vi "logForceActuatorSafetyCheck.vi"(8 "error in (no error)":errorcluster, 10 "EventForceActuatorSafetyChecks":T1, 11 "M1M3SAL in":refnum<class "M1M3SAL.lvclass">) -> (0 "error out":errorcluster, 3 "M1M3SAL out":refnum<class "M1M3SAL.lvclass">)   [LabVIEW 2016, in "M1M3SupportCommunicator.lvlib" / "M1M3SAL.lvclass"]
uses:
  M1M3SAL.lvclass
  DataTypes/Topics/EventForceActuatorSafetyChecks.ctl
  DataTypes/Topics/Parts/Timestamp.ctl
  DataTypes/MessageHeader.ctl
  DataTypes/MessageTypes.ctl
  DataTypes/MessageTopics.ctl
  Common_RT_Utilities/U8ArrayBuilderAutoIndexing/U8ArrayBuilderAutoIndexing.lvclass
  M1M3SupportCommunicator.lvlib
  DataTypes/Topics/M1M3SupportTopics.lvlib
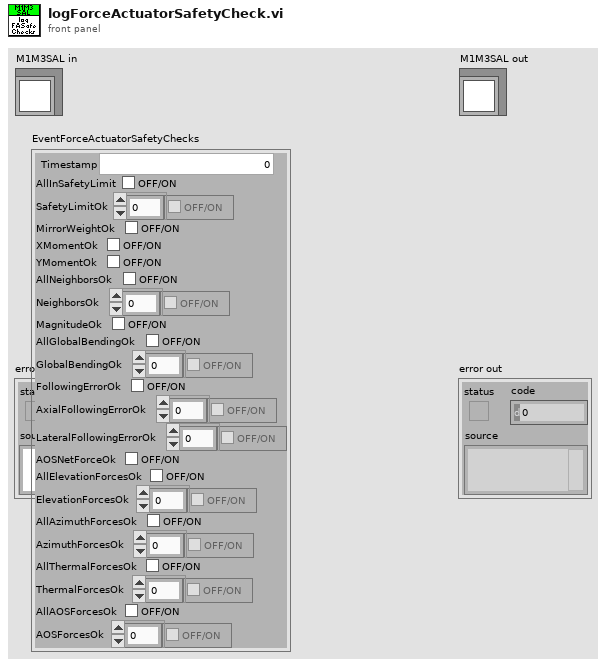
[diagram p1: front panel]
types:
  T1 = typedef "M1M3SupportTopics.lvlib/EventForceActuatorSafetyChecks.ctl" = cluster{"Timestamp":T2, "AllInSafetyLimit":bool, "SafetyLimitOk":bool[], "MirrorWeightOk":bool, "XMomentOk":bool, "YMomentOk":bool, "AllNeighborsOk":bool, "NeighborsOk":bool[], "MagnitudeOk":bool, "AllGlobalBendingOk":bool, "GlobalBendingOk":bool[], "FollowingErrorOk":bool, "AxialFollowingErrorOk":bool[], "LateralFollowingErrorOk":bool[], "AOSNetForceOk":bool, "AllElevationForcesOk":bool, "ElevationForcesOk":bool[], "AllAzimuthForcesOk":bool, "AzimuthForcesOk":bool[], "AllThermalForcesOk":bool, "ThermalForcesOk":bool[], "AllAOSForcesOk":bool, "AOSForcesOk":bool[]}
  T2 = typedef "M1M3SupportTopics.lvlib/Timestamp.ctl" = dbl
  T3 = typedef "M1M3SupportCommunicator.lvlib/MessageHeader.ctl" = cluster{"Type":T4, "Topic":T5, "Size":i32}
  T4 = typedef "M1M3SupportCommunicator.lvlib/MessageTypes.ctl" = enum8{"None", "PutSample", "GetNextSample", "LogEvent", "GetEvent", "IssueCommand", "CommandId", "WaitForCompletion", "AcceptCommand", "AckCommand"}
  T5 = typedef "M1M3SupportCommunicator.lvlib/MessageTopics.ctl" = enum8{"None", "ForceActuatorData", "MirrorForceData", "HardpointData", "AirData", "DynamicData", "FPGAData", "IMSData", "ForceActuatorStatus", "ElevationData", "HardpointStatus", "HardpointActuatorChase", "AirStatus", "ForceActuatorSafetyChecks", "ForceActuatorTest", "ActuatorBroadcastCounter", "StatusChecks", "CellChecks", "HardpointActuatorBreakaway", "RaiseMirrorComplete", "ILCCommunication", "ElevationAngleChecks", "DetailedState", "ServoLoops", "ForceActuatorInfo", "LowerMirrorComplete", "HardpointActuatorInfo", "SettingsApplied", "ErrorCode", "StartupChecks", "SummaryState", "SettingVersions", "ActuatorTestStatus", "AppliedSettingsMatchStart", "Enable", "EnterMaintenance", "Standby", "AbortLowerM1M3", "ApplyAberrationByForces", "ApplyAOSCorrectionByBendingModes", "ClearAOSCorrection", "Start", "RaiseM1M3", "TestForceActuator", "LowerM1M3", "ApplyAOSCorrectionByForces", "Disable", "ApplyAberationByBendingMode", "TestHardpoint", "ManipulateM1M3", "ClearAberration", "Exit", "TestAir", "AbortRaiseM1M3", "MoveHardpointActuators", "ExitMaintenance", "Shutdown"}
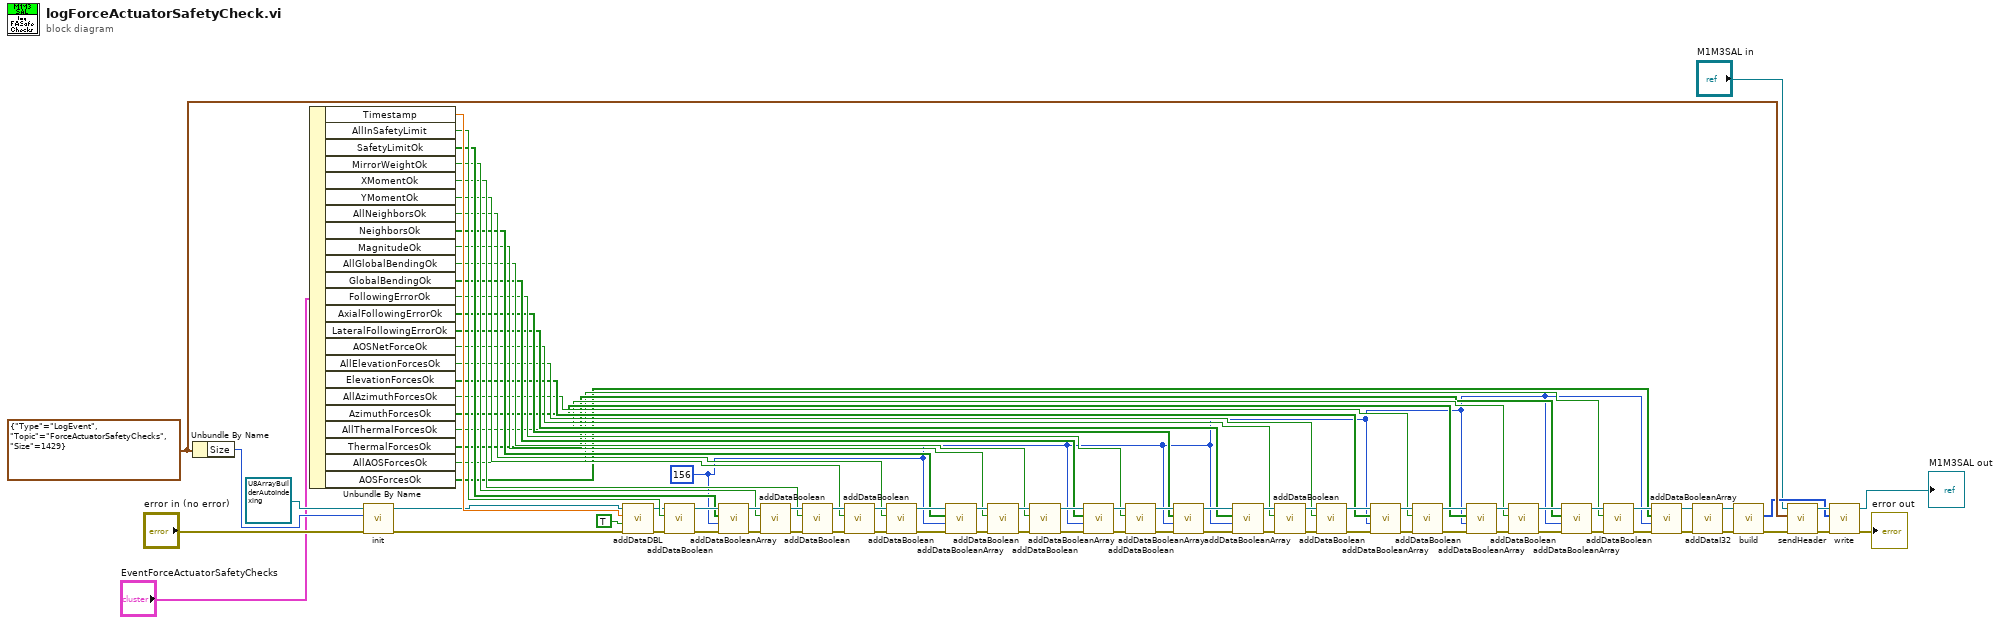
[diagram p0: block diagram]
diagram:
  w1 = 156 ("Length")
  w86 = T3 {"Type"=enum."LogEvent", "Topic"=enum."ForceActuatorSafetyChecks", "Size"=1429} ("MessageHeader")
  n1 = Unbundle By Name(w86) -> ("Size"=w85:i32)
  n2 = Unbundle By Name("EventForceActuatorSafetyChecks") -> ("Timestamp"=w76:T2, "AllInSafetyLimit"=w29:bool, "SafetyLimitOk"=w28:bool[], "MirrorWeightOk"=w27:bool, "XMomentOk"=w26:bool, "YMomentOk"=w25:bool, "AllNeighborsOk"=w24:bool, "NeighborsOk"=w23:bool[], "MagnitudeOk"=w22:bool, "AllGlobalBendingOk"=w21:bool, "GlobalBendingOk"=w20:bool[], "FollowingErrorOk"=w19:bool, "AxialFollowingErrorOk"=w18:bool[], "LateralFollowingErrorOk"=w17:bool[], "AOSNetForceOk"=w16:bool, "AllElevationForcesOk"=w15:bool, "ElevationForcesOk"=w14:bool[], "AllAzimuthForcesOk"=w13:bool, "AzimuthForcesOk"=w12:bool[], "AllThermalForcesOk"=w11:bool, "ThermalForcesOk"=w10:bool[], "AllAOSForcesOk"=w9:bool, "AOSForcesOk"=w8:bool[])
  n3 = call "init.vi"("error in (no error)"="error in (no error)", "Size"=w85, "U8ArrayBuilderAutoIndexing in"=refnum<class "U8ArrayBuilderAutoIndexing.lvclass"> refnum ("RTUtilities.lvlib:U8ArrayBuilderAutoIndexing.lvclass")) -> ("error out"=w73:errorcluster, "U8ArrayBuilderAutoIndexing out"=w75:refnum<class "U8ArrayBuilderAutoIndexing.lvclass">)  [unwired: 7 in]
  n4 = call "addDataDBL.vi"("error in (no error)"=w73, "OverrideSwapBytes"=TRUE, "Data"=w76, "U8ArrayBuilderAutoIndexing in"=w75) -> ("error out"=w6:errorcluster, "U8ArrayBuilderAutoIndexing out"=w7:refnum<class "U8ArrayBuilderAutoIndexing.lvclass">)  [unwired: 6 in]
  n5 = call "addDataBoolean.vi"("error in (no error)"=w6, "Data"=w29, "U8ArrayBuilderAutoIndexing in"=w7) -> ("error out"=w34:errorcluster, "U8ArrayBuilderAutoIndexing out"=w35:refnum<class "U8ArrayBuilderAutoIndexing.lvclass">)  [unwired: 7 in]
  n6 = call "addDataBooleanArray.vi"("error in (no error)"=w34, "Length"=w1, "Data"=w28, "U8ArrayBuilderAutoIndexing in"=w35) -> ("error out"=w71:errorcluster, "U8ArrayBuilderAutoIndexing out"=w70:refnum<class "U8ArrayBuilderAutoIndexing.lvclass">)  [unwired: 6 in]
  n7 = call "addDataBoolean.vi"("error in (no error)"=w71, "Data"=w27, "U8ArrayBuilderAutoIndexing in"=w70) -> ("error out"=w69:errorcluster, "U8ArrayBuilderAutoIndexing out"=w68:refnum<class "U8ArrayBuilderAutoIndexing.lvclass">)  [unwired: 7 in]
  n8 = call "addDataBoolean.vi"("error in (no error)"=w69, "Data"=w26, "U8ArrayBuilderAutoIndexing in"=w68) -> ("error out"=w67:errorcluster, "U8ArrayBuilderAutoIndexing out"=w66:refnum<class "U8ArrayBuilderAutoIndexing.lvclass">)  [unwired: 7 in]
  n9 = call "addDataBoolean.vi"("error in (no error)"=w67, "Data"=w25, "U8ArrayBuilderAutoIndexing in"=w66) -> ("error out"=w65:errorcluster, "U8ArrayBuilderAutoIndexing out"=w64:refnum<class "U8ArrayBuilderAutoIndexing.lvclass">)  [unwired: 7 in]
  n10 = call "addDataBoolean.vi"("error in (no error)"=w65, "Data"=w24, "U8ArrayBuilderAutoIndexing in"=w64) -> ("error out"=w63:errorcluster, "U8ArrayBuilderAutoIndexing out"=w62:refnum<class "U8ArrayBuilderAutoIndexing.lvclass">)  [unwired: 7 in]
  n11 = call "addDataBooleanArray.vi"("error in (no error)"=w63, "Length"=w1, "Data"=w23, "U8ArrayBuilderAutoIndexing in"=w62) -> ("error out"=w61:errorcluster, "U8ArrayBuilderAutoIndexing out"=w60:refnum<class "U8ArrayBuilderAutoIndexing.lvclass">)  [unwired: 6 in]
  n12 = call "addDataBoolean.vi"("error in (no error)"=w61, "Data"=w22, "U8ArrayBuilderAutoIndexing in"=w60) -> ("error out"=w59:errorcluster, "U8ArrayBuilderAutoIndexing out"=w58:refnum<class "U8ArrayBuilderAutoIndexing.lvclass">)  [unwired: 7 in]
  n13 = call "addDataBoolean.vi"("error in (no error)"=w59, "Data"=w21, "U8ArrayBuilderAutoIndexing in"=w58) -> ("error out"=w57:errorcluster, "U8ArrayBuilderAutoIndexing out"=w56:refnum<class "U8ArrayBuilderAutoIndexing.lvclass">)  [unwired: 7 in]
  n14 = call "addDataBooleanArray.vi"("error in (no error)"=w57, "Length"=w1, "Data"=w20, "U8ArrayBuilderAutoIndexing in"=w56) -> ("error out"=w32:errorcluster, "U8ArrayBuilderAutoIndexing out"=w33:refnum<class "U8ArrayBuilderAutoIndexing.lvclass">)  [unwired: 6 in]
  n15 = call "addDataBoolean.vi"("error in (no error)"=w32, "Data"=w19, "U8ArrayBuilderAutoIndexing in"=w33) -> ("error out"=w55:errorcluster, "U8ArrayBuilderAutoIndexing out"=w54:refnum<class "U8ArrayBuilderAutoIndexing.lvclass">)  [unwired: 7 in]
  n16 = call "addDataBooleanArray.vi"("error in (no error)"=w55, "Length"=w1, "Data"=w18, "U8ArrayBuilderAutoIndexing in"=w54) -> ("error out"=w53:errorcluster, "U8ArrayBuilderAutoIndexing out"=w52:refnum<class "U8ArrayBuilderAutoIndexing.lvclass">)  [unwired: 6 in]
  n17 = call "addDataBooleanArray.vi"("error in (no error)"=w53, "Length"=w1, "Data"=w17, "U8ArrayBuilderAutoIndexing in"=w52) -> ("error out"=w51:errorcluster, "U8ArrayBuilderAutoIndexing out"=w50:refnum<class "U8ArrayBuilderAutoIndexing.lvclass">)  [unwired: 6 in]
  n18 = call "addDataBoolean.vi"("error in (no error)"=w51, "Data"=w16, "U8ArrayBuilderAutoIndexing in"=w50) -> ("error out"=w49:errorcluster, "U8ArrayBuilderAutoIndexing out"=w48:refnum<class "U8ArrayBuilderAutoIndexing.lvclass">)  [unwired: 7 in]
  n19 = call "addDataBoolean.vi"("error in (no error)"=w49, "Data"=w15, "U8ArrayBuilderAutoIndexing in"=w48) -> ("error out"=w47:errorcluster, "U8ArrayBuilderAutoIndexing out"=w46:refnum<class "U8ArrayBuilderAutoIndexing.lvclass">)  [unwired: 7 in]
  n20 = call "addDataBooleanArray.vi"("error in (no error)"=w47, "Length"=w1, "Data"=w14, "U8ArrayBuilderAutoIndexing in"=w46) -> ("error out"=w45:errorcluster, "U8ArrayBuilderAutoIndexing out"=w44:refnum<class "U8ArrayBuilderAutoIndexing.lvclass">)  [unwired: 6 in]
  n21 = call "addDataBoolean.vi"("error in (no error)"=w45, "Data"=w13, "U8ArrayBuilderAutoIndexing in"=w44) -> ("error out"=w43:errorcluster, "U8ArrayBuilderAutoIndexing out"=w42:refnum<class "U8ArrayBuilderAutoIndexing.lvclass">)  [unwired: 7 in]
  n22 = call "addDataBooleanArray.vi"("error in (no error)"=w43, "Length"=w1, "Data"=w12, "U8ArrayBuilderAutoIndexing in"=w42) -> ("error out"=w41:errorcluster, "U8ArrayBuilderAutoIndexing out"=w40:refnum<class "U8ArrayBuilderAutoIndexing.lvclass">)  [unwired: 6 in]
  n23 = call "addDataBoolean.vi"("error in (no error)"=w41, "Data"=w11, "U8ArrayBuilderAutoIndexing in"=w40) -> ("error out"=w39:errorcluster, "U8ArrayBuilderAutoIndexing out"=w38:refnum<class "U8ArrayBuilderAutoIndexing.lvclass">)  [unwired: 7 in]
  n24 = call "addDataBooleanArray.vi"("error in (no error)"=w39, "Length"=w1, "Data"=w10, "U8ArrayBuilderAutoIndexing in"=w38) -> ("error out"=w30:errorcluster, "U8ArrayBuilderAutoIndexing out"=w31:refnum<class "U8ArrayBuilderAutoIndexing.lvclass">)  [unwired: 6 in]
  n25 = call "addDataBoolean.vi"("error in (no error)"=w30, "Data"=w9, "U8ArrayBuilderAutoIndexing in"=w31) -> ("error out"=w37:errorcluster, "U8ArrayBuilderAutoIndexing out"=w36:refnum<class "U8ArrayBuilderAutoIndexing.lvclass">)  [unwired: 7 in]
  n26 = call "addDataBooleanArray.vi"("error in (no error)"=w37, "Length"=w1, "Data"=w8, "U8ArrayBuilderAutoIndexing in"=w36) -> ("error out"=w5:errorcluster, "U8ArrayBuilderAutoIndexing out"=w4:refnum<class "U8ArrayBuilderAutoIndexing.lvclass">)  [unwired: 6 in]
  n27 = call "addDataI32.vi"("error in (no error)"=w5, "U8ArrayBuilderAutoIndexing in"=w4) -> ("error out"=w2:errorcluster, "U8ArrayBuilderAutoIndexing out"=w3:refnum<class "U8ArrayBuilderAutoIndexing.lvclass">)  [unwired: 8 in]
  n28 = call "build.vi"("error in (no error)"=w2, "U8ArrayBuilderAutoIndexing in"=w3) -> ("error out"=w82:errorcluster, "Array"=w83:u8[])  [unwired: 7 in, 1 out]
  n29 = call "sendHeader.vi"("error in (no error)"=w82, "MessageHeader"=w86, "M1M3SAL in"="M1M3SAL in") -> ("error out"=w81:errorcluster, "M1M3SAL out"=w84:refnum<class "M1M3SAL.lvclass">)  [unwired: 7 in]
  n30 = call "write.vi"("error in (no error)"=w81, "Data"=w83, "M1M3SAL in"=w84) -> ("error out"=→"error out":errorcluster, "M1M3SAL out"=→"M1M3SAL out":refnum<class "M1M3SAL.lvclass">)  [unwired: 7 in]
